vi "main.vi"() -> ()   [LabVIEW 2018]
uses:
  <vilib>/Waveform/WDTOps.llb/WDT Get Waveform Subset DBL.vi
  <vilib>/express/express analysis/Spectral/Block/exnSpectralBlock spectral measurements RMS poly.vi
  <vilib>/express/express analysis/Spectral/Block/exnSpectralBlock spectral measurements RMS DDT.vi
  <vilib>/express/express analysis/Spectral/XNode/ExpressSpectralMeasurementsBlockNode.xnode
panel:
  out "ampl":dynamicdata(graph)
  in  "odstupanje ref":dbl
  out "IQ 2MHz  spektar":dynamicdata(graph)
  out "izolovana povorka":waveform(dbl)(graph)
  out "IQ 2MHz":dynamicdata(graph)
  out "spektar izolovane povorke":cluster{"f0":dbl, "df":dbl, "magnitude":dbl[]}(graph)
  in  "dopler f":dbl format="%#.6f"
  out "I pre filtra":dynamicdata(graph)
  in  "ampl suma ulaza":dbl
  in  "amplituda suma ref":dbl
  in  "amplituda \nnoseceg":dbl
  in  "frekv ref":dbl
  in  "amplituda \nglavnog":dbl
  in  "pocetna faza\nglavnog":dbl
  out "Waveform Graph":dynamicdata(graph)
  out "ulazni_spektar":dynamicdata(graph)
  out "Ulazni signal":dynamicdata(graph)
  out "Q grana":dynamicdata(graph)
  out "REF 30MHz cos":waveform(dbl)(graph)
  out "spektarIQmod 2":dynamicdata(graph)
  out "I grana":dynamicdata(graph)
  out "spektar REF sin":dynamicdata(graph)
  out "REF 30MHZ sin":dynamicdata(graph)
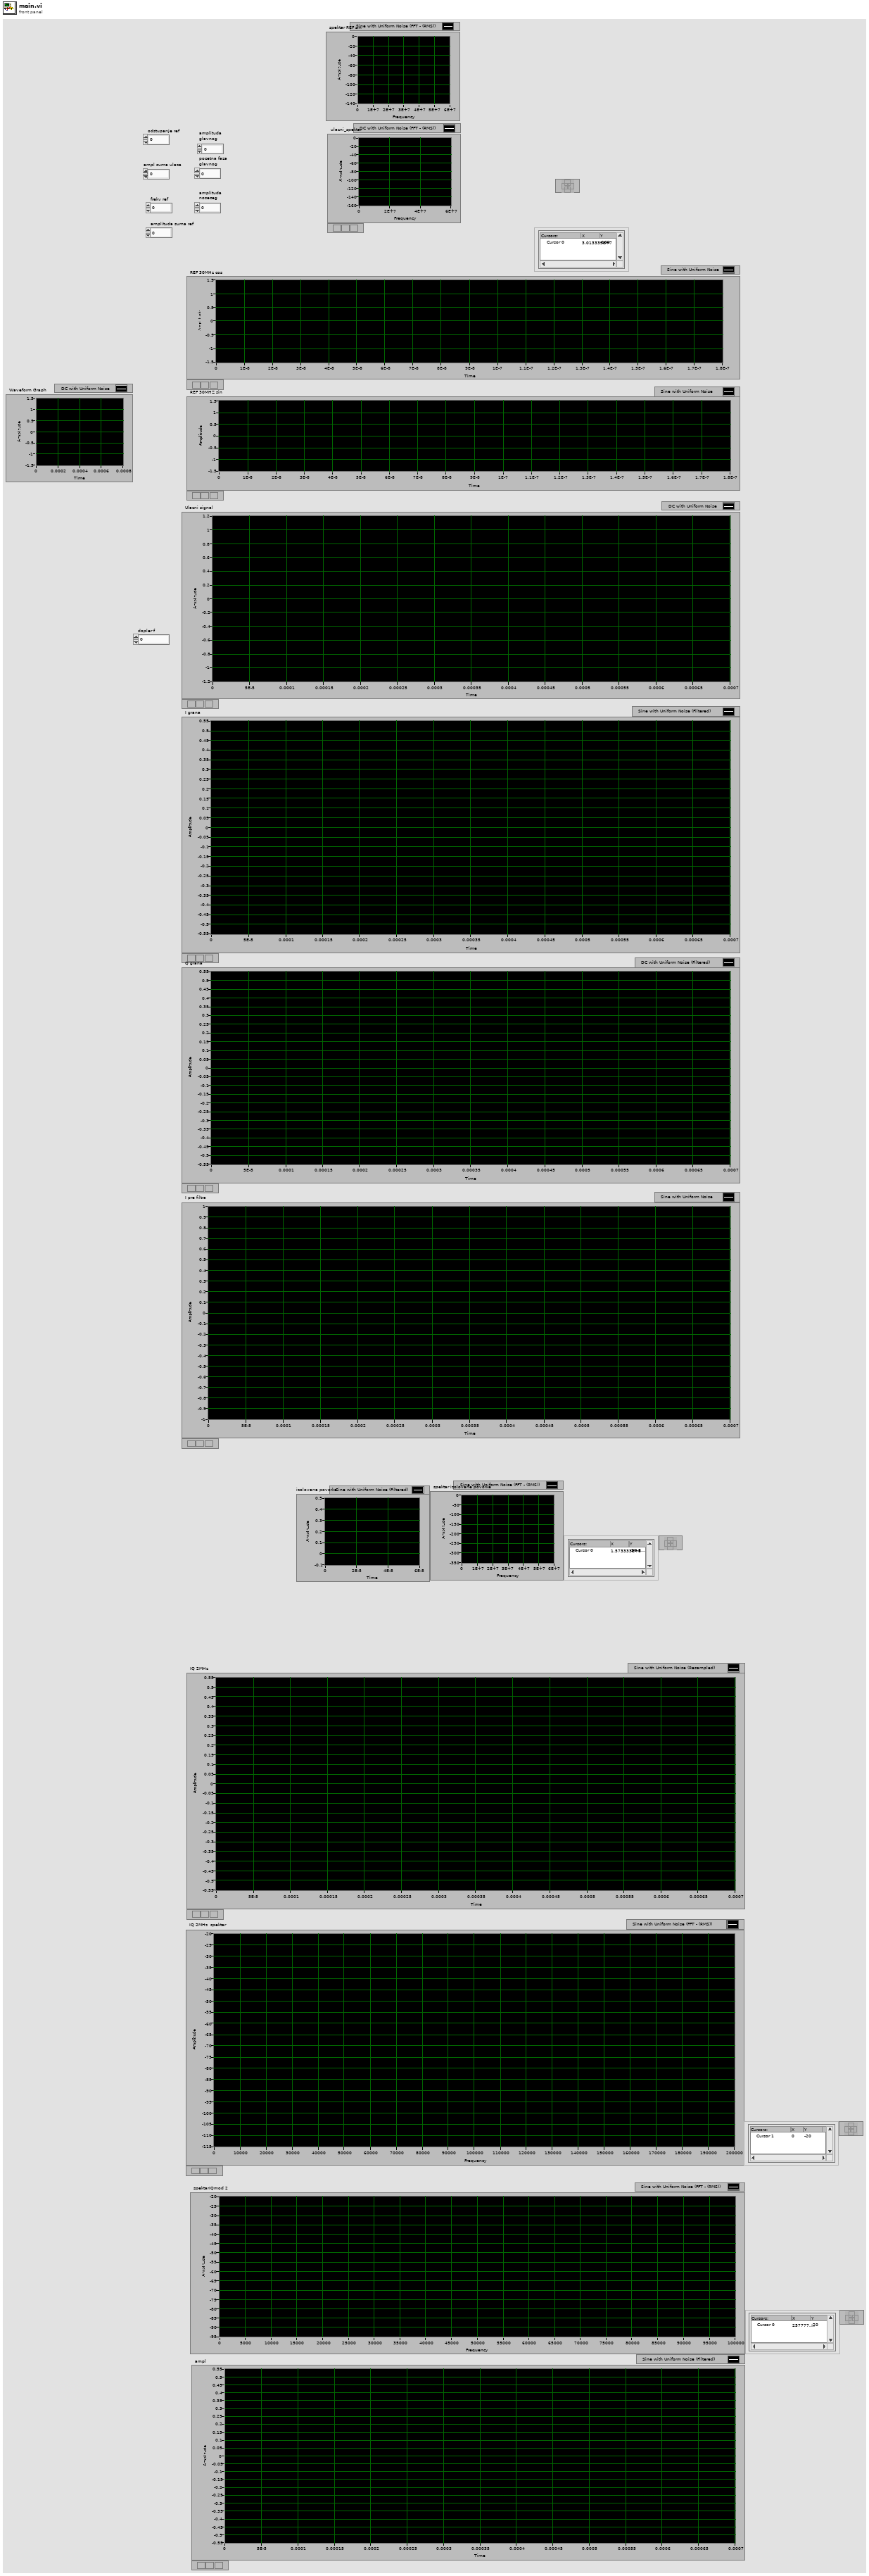
[diagram p1: front panel]
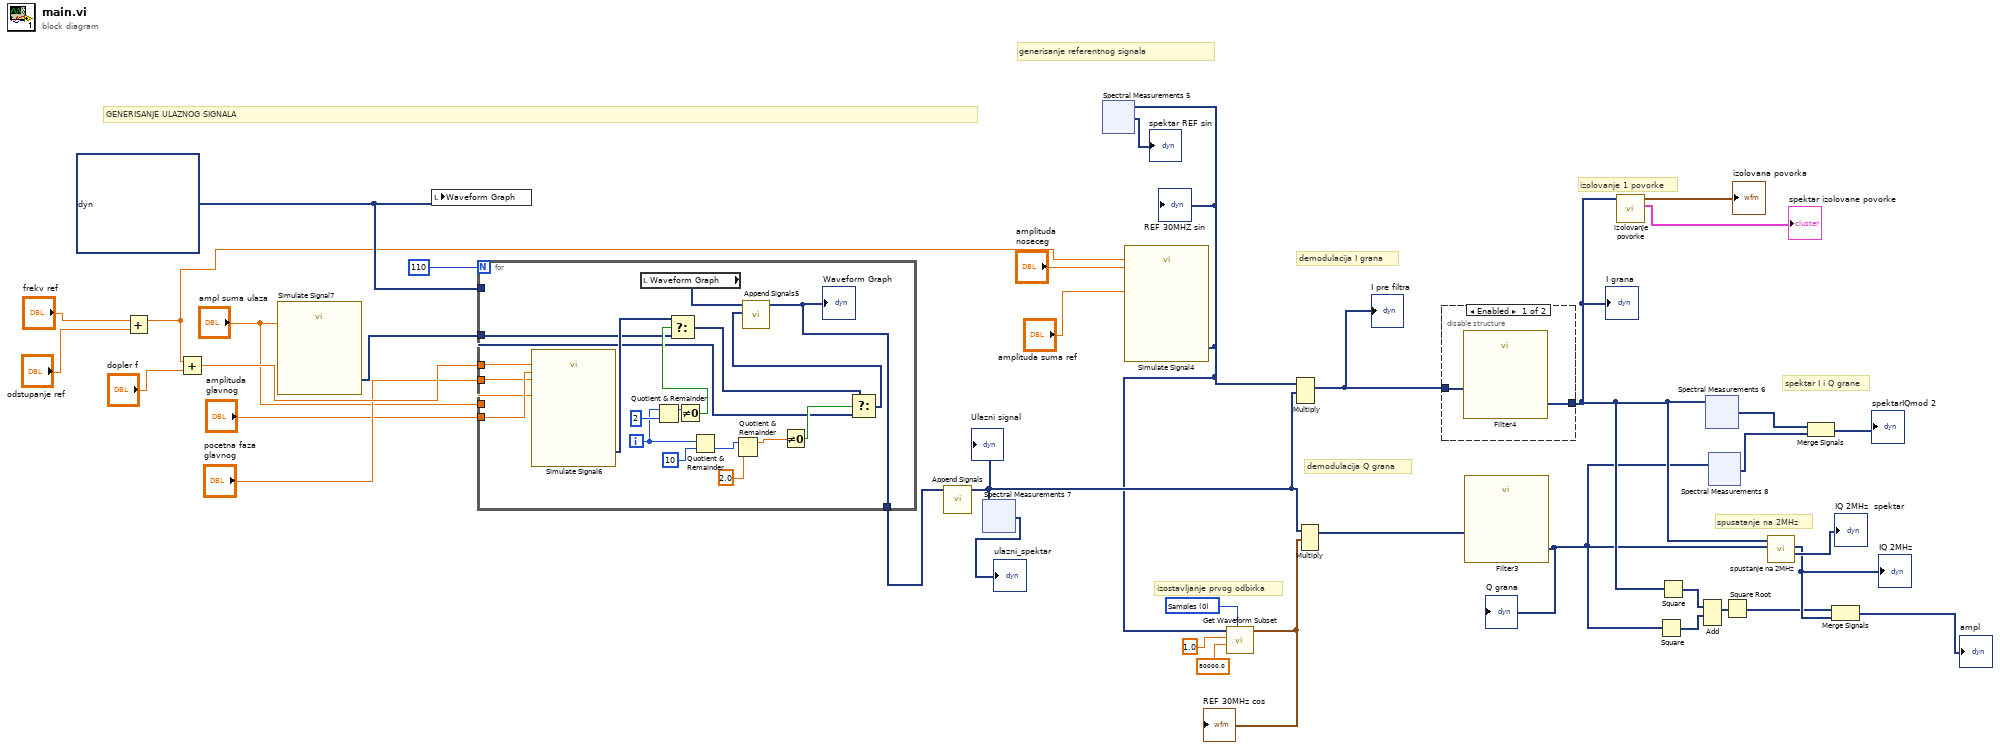
[diagram p0: block diagram]
diagram:
  w20 = u16 0 items=["Samples", "Relative Time"] ("start/duration format")
  w35 = dynamicdata [] ("Waveform Graph")
  # "generisanje referentnog signala"
  # "izolovanje 1 povorke"
  # "spusatanje na 2MHz"
  # "spektar I i Q grane"
  # "izostavljanje prvog odbirka"
  # "demodulacija Q grana"
  # "demodulacija I grana"
  # "GENERISANJE ULAZNOG SIGNALA"
  n1 = Add(x="frekv ref", y="odstupanje ref") -> (x+y=w9:dbl)
  n2 = Add(x=w9, y="dopler f") -> (x+y=w24:dbl)
  n3 = call "Simulate Signal7"("Noise amplitude"="ampl suma ulaza") -> ("DC with Uniform Noise"=w25:dynamicdata)  [unwired: 13 in, 1 out]
  n4 = local write "Waveform Graph"(w35) -> ()
  n5 = for {
    N: 110 -> [_]
    tunnel: w35 -> [_]
    tunnel: [w53] -> w29
    tunnel: w25 -> [w39]
    tunnel: w24 -> [w47]
    tunnel: "pocetna faza\nglavnog" -> [w45]
    tunnel: "amplituda \nglavnog" -> [w46]
    tunnel: "ampl suma ulaza" -> [w44]
    i -> [w48]
    n6 = call "Simulate Signal6"("Frequency"=w47, "Amplitude"=w46, "Phase"=w45, "Noise amplitude"=w44) -> ("Sine with Uniform Noise"=w43:dynamicdata)  [unwired: 10 in, 1 out]
    n7 = local read "Waveform Graph"() -> (w57:dynamicdata)
    n8 = Quotient & Remainder(x=w48, y=2) -> (x-y*floor(x/y)=w55:i32)  [unwired: 1 out]
    n9 = Not Equal To 0?(x=w55) -> (x != 0?=w54:bool)
    n10 = Select(t=w43, s=w54, f=w39) -> (s? t:f=w50:dynamicdata)
    n11 = Quotient & Remainder(x=w48, y=10) -> (floor(x/y)=w41:i32)  [unwired: 1 out]
    n12 = Quotient & Remainder(x=w41, y=2.0) -> (x-y*floor(x/y)=w40:dbl)  [unwired: 1 out]
    n13 = Not Equal To 0?(x=w40) -> (x != 0?=w51:bool)
    n14 = Select(t=w50, s=w51, f=w39) -> (s? t:f=w49:dynamicdata)
    n15 = call "Append Signals5"("Input Signal B"=w49, "Input Signal A"=w57) -> ("Appended Signals"=w53:dynamicdata)  [unwired: 8 in, 1 out]
    "Waveform Graph" <- w53
  }
  n16 = call "Append Signals"("Input Signal A"=w29) -> ("Appended Signals"=w23:dynamicdata)  [unwired: 9 in, 1 out]
  "Ulazni signal" <- w23
  n17 = xnode "Spectral Measurements 7"("Signals"=w23) -> ("FFT - (RMS)"=→"ulazni_spektar":dynamicdata)  [unwired: 1 in, 2 out]
  n18 = call "Simulate Signal4"("Frequency"=w9, "Amplitude"="amplituda \nnoseceg", "Noise amplitude"="amplituda suma ref") -> ("Sine with Uniform Noise"=w22:dynamicdata)  [unwired: 11 in, 1 out]
  "REF 30MHZ sin" <- w22
  n19 = xnode "Spectral Measurements 5"("Signals"=w22) -> ("FFT - (RMS)"=→"spektar REF sin":dynamicdata)  [unwired: 1 in, 2 out]
  n20 = call-poly <vilib>:"Get Waveform Subset.vi"("start/duration format"=w20, "duration"=80000.0, "start samples/time"=1.0 ("actual duration"), "waveform in"=w22) -> ("waveform out"=w21:waveform(dbl))  [unwired: 2 in, 3 out]
  "REF 30MHz cos" <- w21
  n21 = Multiply(1:w23, 2:w22) -> (0:w27:dynamicdata)  [unwired: 1 in, 1 out]
  "I pre filtra" <- w27
  n22 = Multiply(1:w21, 2:w23) -> (0:w28:dynamicdata)  [unwired: 1 in, 1 out]
  n23 = disable-structure shown="Enabled" {
    disable-tunnel: w27 -> [w59 w60]
    disable-tunnel: [w58 w60] -> w8
    frame Enabled {
      n24 = call "Filter4"("Signal"=w59) -> ("Filtered Signal"=w58:dynamicdata)  [unwired: 9 in, 1 out]
    }
    frame Disabled {
    }
  }
  "I grana" <- w8
  n25 = call "Filter3"("Signal"=w28) -> ("Filtered Signal"=w7:dynamicdata)  [unwired: 9 in, 1 out]
  "Q grana" <- w7
  n26 = call "izolovanje povorke.vi"("Filtered Signal"=w8) -> ("spektar izolovane povorke"=→"spektar izolovane povorke":cluster{"f0":dbl, "df":dbl, "magnitude":dbl[]}, "izolovana povorka"=→"izolovana povorka":waveform(dbl))  [unwired: 9 in]
  n27 = Square(x=w7) -> (x^2=w5:dynamicdata)
  n28 = Square(x=w8) -> (x^2=w6:dynamicdata)
  n29 = Add(1:w5, 2:w6) -> (0:w2:dynamicdata)  [unwired: 1 in, 1 out]
  n30 = xnode ("Spectral Measurements 6")("Signals"=w8) -> ("FFT - (RMS)"=w37:dynamicdata)  [unwired: 1 in, 2 out]
  n31 = xnode ("Spectral Measurements 8")("Signals"=w7) -> ("FFT - (RMS)"=w30:dynamicdata)  [unwired: 1 in, 2 out]
  n32 = Square Root(x=w2) -> (sqrt(x)=w1:dynamicdata)
  n33 = call "spustanje na 2MHz.vi"("Filtered Signal 2"=w7, "Filtered Signal"=w8) -> ("IQ 2MHz  spektar"=→"IQ 2MHz  spektar":dynamicdata, "IQ 2MHz"=w3:dynamicdata)  [unwired: 6 in, 2 out]
  "IQ 2MHz" <- w3
  n34 = Merge Signals(w37, w30) -> (→"spektarIQmod 2":dynamicdata)
  n35 = Merge Signals(w1, w3) -> (→"ampl":dynamicdata)
